vi "Shutdown Common.vi"(8 "error in (no error)":errorcluster, 11 "Actor in":refnum<class "Actor.lvclass">) -> (0 "error out":errorcluster, 3 "Actor out":refnum<class "Actor.lvclass">)   [LabVIEW 2015, in "Actor.lvclass"]
uses:
  Actor.lvclass
  Actor.lvclass/Actor.ctl
  Utility/Utility.lvlib
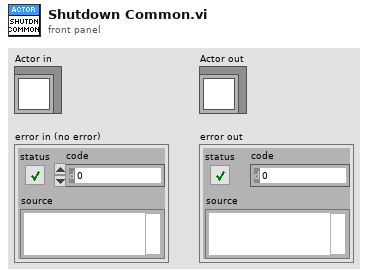
[diagram p1: front panel]
types:
  T1 = typedef "Actor.lvclass/Update User Event.ctl" = refnum<user-event>
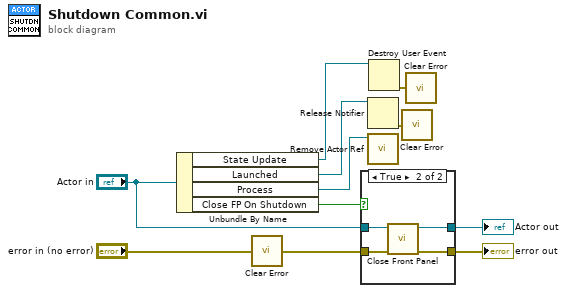
[diagram p0: block diagram]
diagram:
  n1 = Unbundle By Name("Actor in") -> ("State Update"=w1:T1, "Launched"=w4:refnum<notifier>, "Process"=w5:refnum<vi>, "Close FP On Shutdown"=w7:bool)
  n2 = call "Clear Error.vi"("error in (no error)"="error in (no error)") -> ("error out"=w6:errorcluster)
  n3 = case shown="True" w7 {
    tunnel: w6 -> [w12 w17]
    tunnel: "Actor in" -> [w13 w16]
    tunnel: [w13 w15] -> w10
    tunnel: [w12 w14] -> w8
    frame False {
    }
    frame True {
      n4 = call-dynamic "Close Front Panel.vi"("error in (no error)"=w17, "Actor in"=w16) -> ("error out"=w14:errorcluster, "Actor out"=w15:refnum<class "Actor.lvclass">)  [unwired: 8 in]
    }
  }
  "Actor out" <- w10
  "error out" <- w8
  n5 = Release Notifier(notifier=w4) -> (error out=w3:errorcluster)  [unwired: 2 in, 2 out]
  n6 = call "Remove Actor Ref.vi"("VI Refnum In"=w5) -> ()  [unwired: 11 in]
  n7 = Destroy User Event(user event=w1) -> (error out=w2:errorcluster)  [unwired: 1 in]
  n8 = call "Clear Error.vi"("error in (no error)"=w3) -> ()  [unwired: 1 out]
  n9 = call "Clear Error.vi"("error in (no error)"=w2) -> ()  [unwired: 1 out]
